vi "CLC_JIO_subBFIC.vi"(7 "pol":u16, 8 "error in":errorcluster, 10 "ele":i32, 11 "com":i32) -> (0 "error out":errorcluster, 3 "standard output":string)   [LabVIEW 2023, in "CLC_JIO_FTDI.lvlib"]
uses:
  CLC_JIO_FTDI.lvlib
panel:
  out "appended path":path
  out "standard error":string
  out "floder?":bool
  # "0:H\n1:V\n2:H+V"
  # "0-15"
  # "0-15"
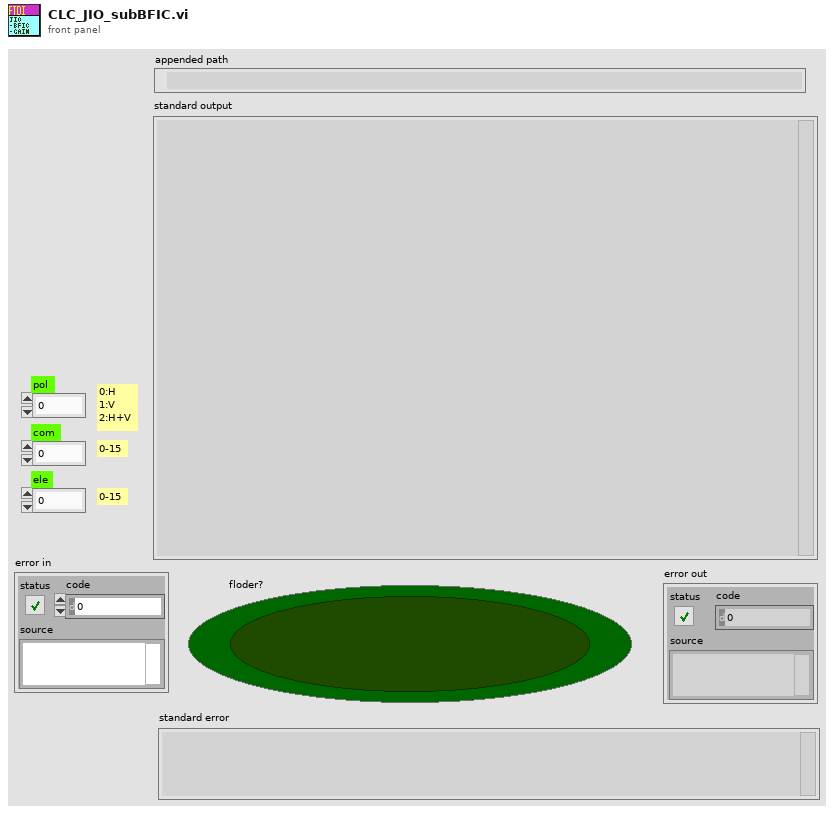
[diagram p1: front panel]
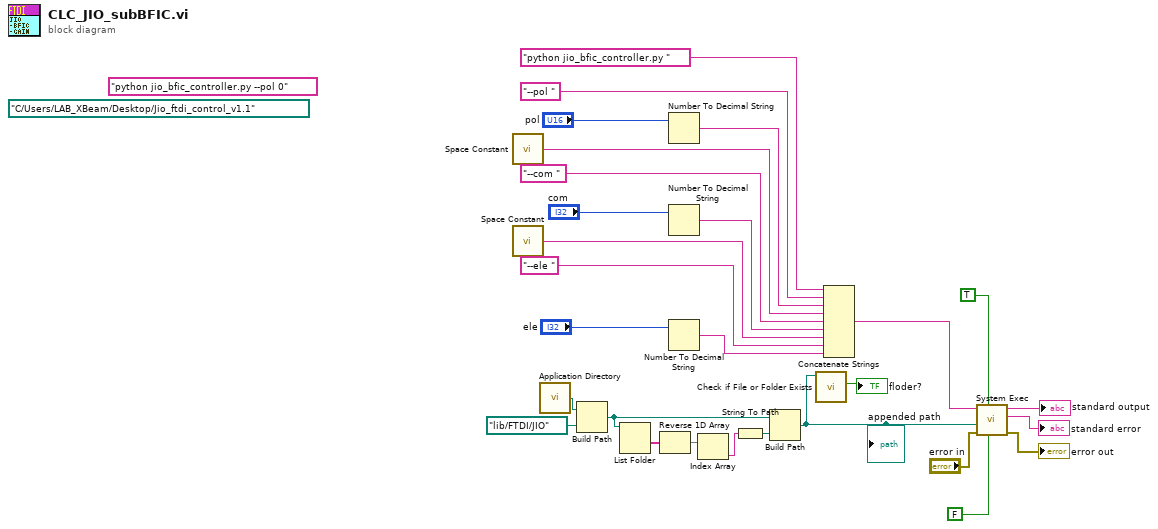
[diagram p0: block diagram]
diagram:
  (unwired) "python jio_bfic_controller.py --pol 0" ("command line")
  (unwired) path "C:/Users/LAB_XBeam/Desktop/Jio_ftdi_control_v1.1" ("working directory")
  n1 = call <vilib>:"Space Constant.vi"() -> ("String"=w7:string)
  n2 = call <vilib>:"Space Constant.vi"() -> ("String"=w11:string)
  n3 = call <vilib>:"Application Directory.vi"() -> ("Application Directory"=w22:path)
  n4 = Build Path(base path=w22, name or relative path=path "lib/FTDI/JIO") -> (appended path=w21:path)
  n5 = List Folder(path=w21) -> (folder names=w27:string[])  [unwired: 3 in, 3 out]
  n6 = Reverse 1D Array(array=w27) -> (reversed array=w26:string[])
  n7 = Number To Decimal String(number="pol") -> (decimal integer string=w16:string)  [unwired: 1 in]
  n8 = Number To Decimal String(number="com") -> (decimal integer string=w13:string)  [unwired: 1 in]
  n9 = Number To Decimal String(number="ele") -> (decimal integer string=w9:string)  [unwired: 1 in]
  n10 = Index Array(array=w26) -> (element=w25:string)  [unwired: 1 in]
  n11 = String To Path(string=w25) -> (path=w24:path)
  n12 = Build Path(base path=w21, name or relative path=w24) -> (appended path=w6:path)
  "appended path" <- w6
  n13 = call <vilib>:"Check if File or Folder Exists.vi"("path"=w6) -> ("file or folder exists?"=→"floder?":bool)  [unwired: 8 in, 2 out]
  n14 = Concatenate Strings("python jio_bfic_controller.py " ("string"), "--pol " ("string"), w16, w7, "--com " ("string"), w13, w11, "--ele " ("string"), w9) -> (w8:string)
  n15 = call <vilib>:"System Exec.vi"("run minimized? (F)"=FALSE, "wait until completion? (T)"=TRUE, "error in (no error)"="error in", "working directory"=w6, "command line"=w8) -> ("error out"=→"error out":errorcluster, "standard error"=→"standard error":string, "standard output"=→"standard output":string)  [unwired: 3 in, 1 out]
